vi "analyzeNonlinearities.vi"(8 "error":errorcluster, 10 "axis":i32, 11 "connection ID":refnum<k5>) -> (0 "error out":errorcluster, 2 "axis_out":i32, 3 "connection ID out":refnum<k5>)   [LabVIEW 2016, in "sen_api.lvlib"]
doc: "Estimates the nonlinearity error for the current device settings without modifying \n any settings. After applying a LUT, this function can be used to determine the effectiveness \n of the applied LUT. The error curve as a function of phase can be retrieved using \n getNonlinearityErrorCurveInPm(). The error list, for example for histogram evaluation, \n can be retrieved using getNonlinearityErrorListInPm(). If the estimation fails, for example \n due to an unstable measurement setup, the previously stored estimation results are not updated. \n In this case, subsequent calls to the corresponding get-functions return the last valid results.\n This function is only available in the \"\"measurement running\"\" state. While the estimation \n is running, the device state changes to \"\"measurement starting\"\". \n Refer to system.getCurrentMode() for state details."
uses:
  sen_api.lvlib
panel:
  out "jsonRespIn":string
  out "JSON-response":string="{\"jsonrpc\":\"2.0\",\"method\":\"\",\"params\":[5,1.245,true,\"name\"],\"id\":\"1\"}"
  out "JSON request":string
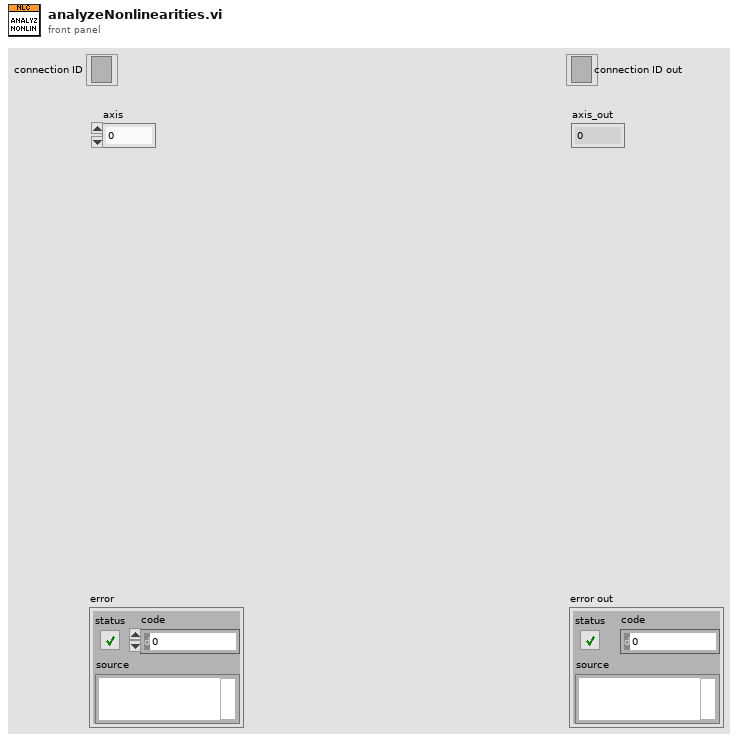
[diagram p1: front panel]
types:
  T1 = cluster{"jsonrpc":string, "method":string, "params":string[], "id":string, "api":i32, "pid":string}
  T2 = enum16{"Standard", "Buffered", "CRLF", "Immediate"}
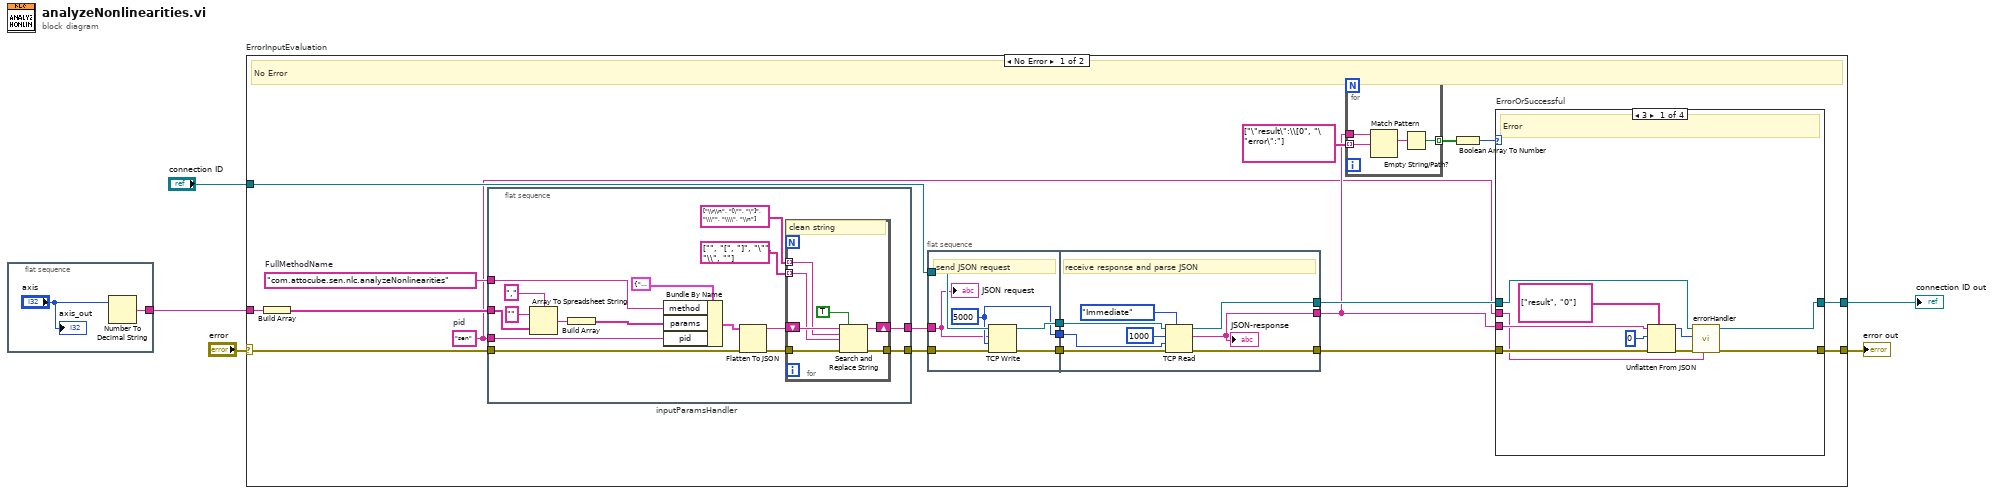
[diagram p0: block diagram]
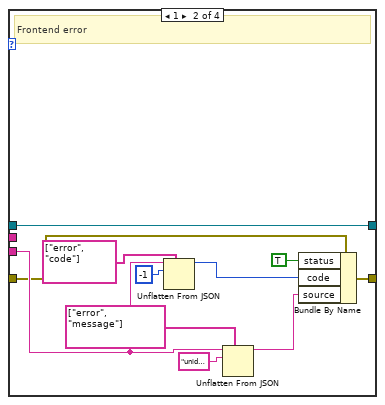
[diagram p2: hidden frame]
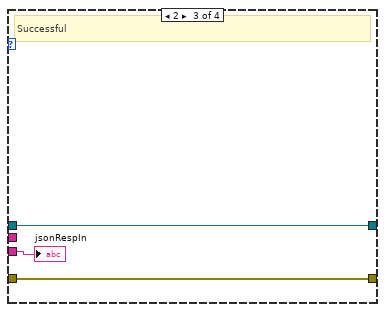
[diagram p3: hidden frame]
diagram:
  n1 = flat-sequence "in_axis" {
    tunnel: [w7] -> w1
    frame #0 {
      n2 = Number To Decimal String(number="axis") -> (decimal integer string=w7:string)  [unwired: 1 in]
      "axis_out" <- "axis"
    }
  }
  n3 = case "ErrorInputEvaluation" shown="No Error" "error" {
    selector: "error" -> [w13 w94]
    tunnel: "connection ID" -> [w23 w95]
    tunnel: [w15 w94] -> w4
    tunnel: [w16 w95] -> w3
    tunnel: w1 -> [w8 _]
    frame No Error {
      w9 = "sen"  # pid
      w14 = "com.attocube.sen.nlc.analyzeNonlinearities"  # FullMethodName
      # "No Error"
      n4 = Build Array ("ParametersArrayString")(w8) -> (w12:string[])
      n5 = flat-sequence "inputParamsHandler" {
        tunnel: [w30] -> w11
        tunnel: w12 -> [w37]
        tunnel: w13 -> [w35]
        tunnel: [w32] -> w10
        tunnel: w14 -> [w38]
        tunnel: w9 -> [w27]
        frame #0 {
          n6 = Array To Spreadsheet String(delimiter (Tab)=",", array=w37, 3:"" ("format string")) -> (spreadsheet string=w40:string)
          n7 = Build Array "Build Array"(w40) -> (w36:string[])
          n8 = Bundle By Name(cluster=T1 {"jsonrpc"="2.0", "method"="com.attocube.amc.res.setRESReadOutFreq", "params"=[], "id"="1", "api"=2, "pid"=""}, "method"=w38, "params"=w36, "pid"=w27) -> (w39:T1)
          n9 = Flatten To JSON(anything=w39, error in (no error)=w35) -> (JSON string=w31:string, 11:w33:errorcluster)  [unwired: 1 in]
          n10 = for {
            tunnel: string[] ["\\r\\n", "[\"", "\"]", "\\\"", "\\\\", "\\n"] ("search string") -> [w46] mode=indexing
            tunnel: string[] ["", "[", "]", "\"", "\\", ""] ("replace string (\"\")") -> [w45] mode=indexing
            shift-right: [w48] -> w30
            shift-left: w31 -> [w47]
            tunnel: w33 -> [w44]
            tunnel: [w43] -> w32
            # "clean string"
            n11 = Search and Replace String(replace all?=TRUE ("replace all? (F)"), input string=w47, search string=w46, replace string=w45, error in=w44) -> (result string=w48:string, error out=w43:errorcluster)  [unwired: 3 in, 2 out]
          }
        }
      }
      n12 = flat-sequence {
        tunnel: w23 -> [w85]
        tunnel: [w83] -> w26
        tunnel: [w84] -> w25
        tunnel: w10 -> [w80]
        tunnel: [w82] -> w24
        tunnel: w11 -> [w81]
        tunnel: [w89] -> w19
        tunnel: w26 -> [w91]
        tunnel: w25 -> [w90]
        tunnel: [w87] -> w18
        tunnel: w24 -> [w88]
        tunnel: [w86] -> w17
        frame #0 {
          w82 = 5000 ("timeout ms (25000)")
          # "send JSON request"
          n13 = TCP Write(connection ID=w85, data in=w81, error in (no error)=w80, 9:w82) -> (connection ID out=w83:refnum<k5>, error out=w84:errorcluster)  [unwired: 1 out]
          "JSON request" <- w81
        }
        frame #1 {
          # "receive response and parse JSON"
          n14 = TCP Read(connection ID=w91, bytes to read=1000, error in (no error)=w90, 7:T2."Immediate" ("mode (standard)"), 9:w88) -> (connection ID out=w89:refnum<k5>, data out=w86:string, error out=w87:errorcluster)
          "JSON-response" <- w86
        }
      }
      n15 = for {
        tunnel: string[] ["\"result\":\\[0", "\"error\":"] ("path") -> [w52] mode=indexing
        tunnel: [w50] -> w21 mode=indexing
        tunnel: w17 -> [w53]
        n16 = Match Pattern(string=w53, regular expression=w52) -> (match substring=w51:string)  [unwired: 1 in, 3 out]
        n17 = Empty String/Path?(string/path=w51) -> (empty?=w50:bool)
      }
      n18 = Boolean Array To Number(Boolean array=w21) -> (number=w20:u32)
      n19 = case "ErrorOrSuccessful" shown="3" w20 {
        tunnel: w17 -> [w57 w66 w75 _]
        tunnel: w19 -> [w61 w64 w77 w79]
        tunnel: [w59 w64 w77 w79] -> w16
        tunnel: [w60 w67 w76 w78] -> w15
        tunnel: w18 -> [w63 w65 w76 w78]
        tunnel: w9 -> [w54 _ _ _]
        frame 3 {
          # "Error"
          n20 = Unflatten From JSON(path=string[] ["result", "0"], JSON string=w57, type and defaults=0, error in (no error)=w63) -> (value=w55:i32, error out=w62:errorcluster)  [unwired: 3 in]
          n21 = call "errorHandler.vi"("pid"=w54, "error in"=w62, "errNbr"=w55, "connection ID"=w61) -> ("error out 2"=w60:errorcluster, "connection ID out"=w59:refnum<k5>)  [unwired: 6 in]
        }
        frame 1 {
          # "Frontend error"
          n22 = Unflatten From JSON(path=string[] ["error", "code"], JSON string=w66, type and defaults=-1) -> (value=w73:i32)  [unwired: 4 in, 1 out]
          n23 = Unflatten From JSON(path=string[] ["error", "message"], JSON string=w66, type and defaults="unidentified error") -> (value=w74:string)  [unwired: 4 in, 1 out]
          n24 = Bundle By Name(cluster=w65, "status"=TRUE, "code"=w73, "source"=w74) -> (w67:errorcluster)
        }
        frame 2 {
          # "Successful"
          "jsonRespIn" <- w75
        }
        frame Default {
          # "NoResponse"
        }
      }
    }
    frame Error {
      # "Error"
    }
  }
  "error out" <- w4
  "connection ID out" <- w3
